vi "Path Get Steam Path.vi"(8 "error in (no error)":errorcluster) -> (0 "error out":errorcluster, 3 "Steam Path":path)   [LabVIEW 2018, in "Main Panel.lvlib" / "Main Panel.lvclass"]
uses:
  Main Panel.lvclass
  <vilib>/registry/registry.llb/Registry RtKey.ctl
  <vilib>/registry/registry.llb/Read Registry Value Simple STR.vi
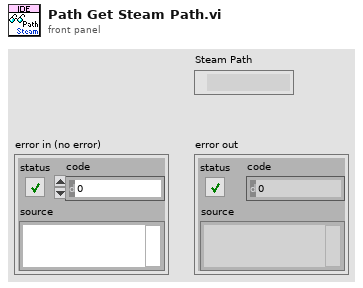
[diagram p1: front panel]
types:
  T1 = typedef "Registry RtKey.ctl" = enum32{"HKEY_CLASSES_ROOT", "HKEY_CURRENT_USER", "HKEY_LOCAL_MACHINE", "HKEY_USERS", "HKEY_PERFORMANCE_DATA", "HKEY_CURRENT_CONFIG", "HKEY_DYN_DATA"}
  T2 = typedef "Registry refnum.ctl" = refnum<k1>
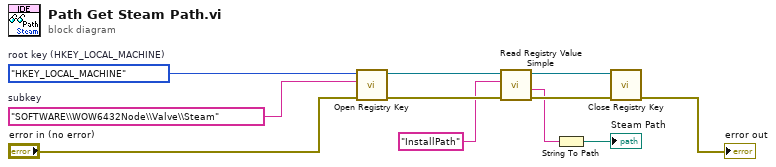
[diagram p0: block diagram]
diagram:
  w8 = "SOFTWARE\\WOW6432Node\\Valve\\Steam"  # subkey
  w9 = Registry_RtKey."HKEY_LOCAL_MACHINE"  # root key (HKEY_LOCAL_MACHINE)
  n1 = call <vilib>:"Open Registry Key.vi"("error in (no error)"="error in (no error)", "subkey"=w8, "root key (HKEY_LOCAL_MACHINE)"=w9) -> ("error out"=w10:errorcluster, "refnum out"=w11:T2)  [unwired: 7 in]
  n2 = call-poly <vilib>:"Read Registry Value Simple.vi"("error in (no error)"=w10, "value"="InstallPath", "refnum"=w11) -> ("error out"=w5:errorcluster, "String/Binary data"=w4:string, "refnum out"=w6:T2)  [unwired: 3 in, 1 out]
  n3 = String To Path(string=w4) -> (path=→"Steam Path":path)
  n4 = call <vilib>:"Close Registry Key.vi"("error in (no error)"=w5, "refnum"=w6) -> ("error out"=→"error out":errorcluster)  [unwired: 5 in]
